vi "Start All Task.vi"(7 "when":timestamp, 8 "error in":errorcluster, 10 "rate":dbl=1000.0 format="%0.2f", 11 "Task in":T1) -> (0 "error out":errorcluster, 3 "Task out":T1)   [LabVIEW 2022 SP3]
uses:
  <vilib>/DAQmx/configure/trigger.llb/DAQmx Start Trigger (Time).vi
  <vilib>/DAQmx/configure/timing.llb/DAQmx Timing (Sample Clock).vi
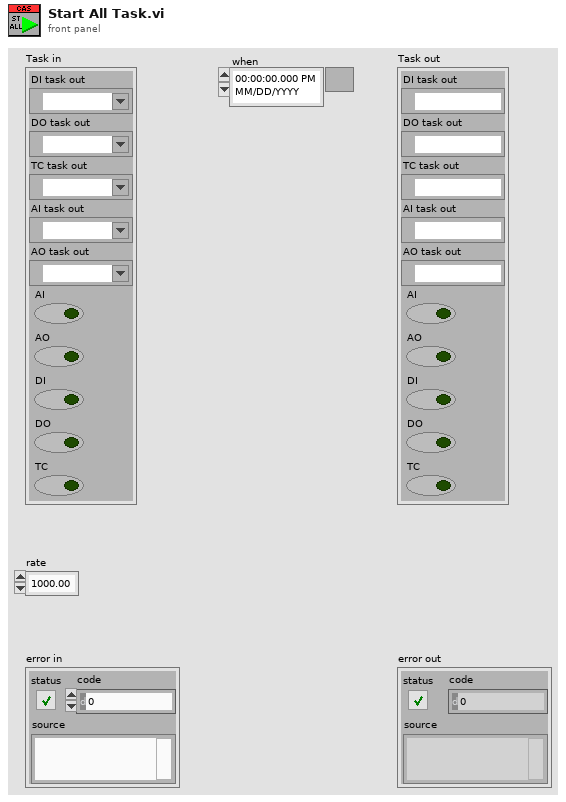
[diagram p1: front panel]
types:
  T1 = cluster{"DI task out":refnum<k21>, "DO task out":refnum<k21>, "TC task out":refnum<k21>, "AI task out":refnum<k21>, "AO task out":refnum<k21>, "AI":bool, "AO":bool, "DI":bool, "DO":bool, "TC":bool}
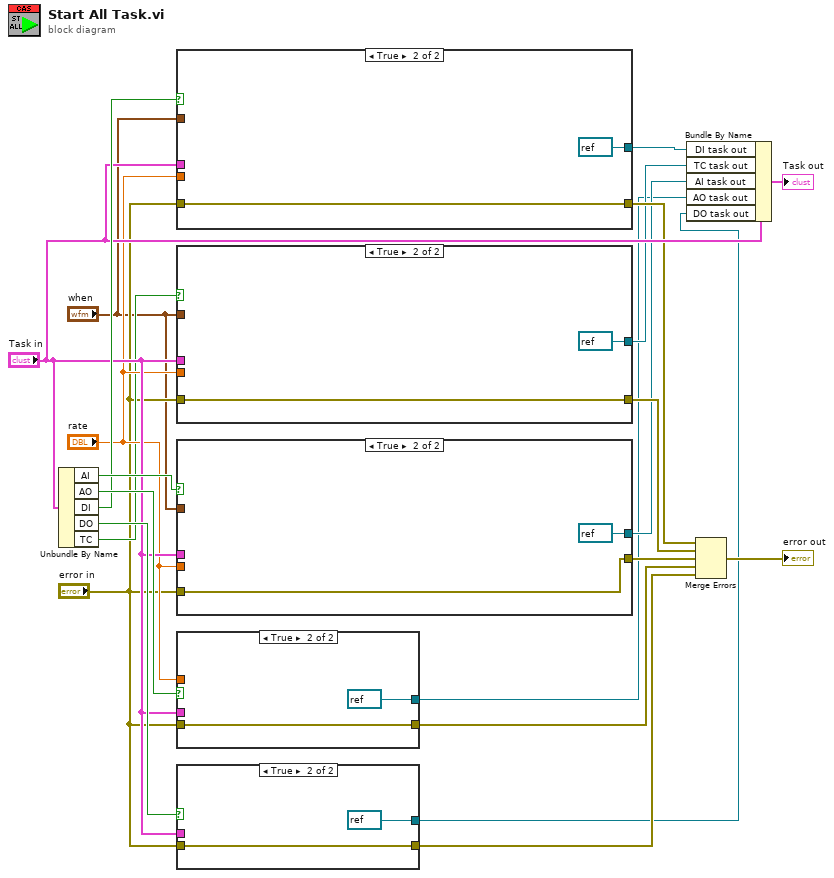
[diagram p0: block diagram]
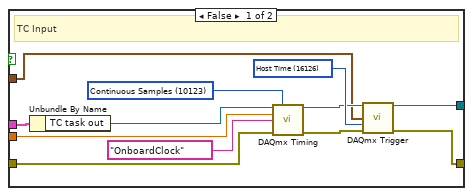
[diagram p2: hidden frame]
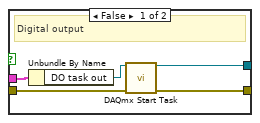
[diagram p3: hidden frame]
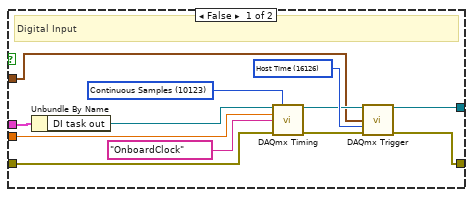
[diagram p4: hidden frame]
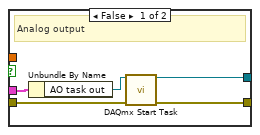
[diagram p5: hidden frame]
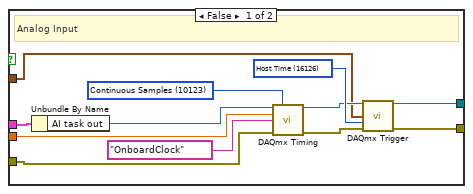
[diagram p6: hidden frame]
diagram:
  n1 = Unbundle By Name("Task in") -> ("AI"=w21:bool, "AO"=w20:bool, "DI"=w19:bool, "DO"=w18:bool, "TC"=w15:bool)
  n2 = case shown="True" w19 {
    tunnel: [w28 w35] -> w13
    tunnel: "rate" -> [w27 _]
    tunnel: "when" -> [w26 _]
    tunnel: "Task in" -> [w23 _]
    tunnel: "error in" -> [w24 w35]
    tunnel: [w22 refnum<k21> refnum ("task out")] -> w7
    frame False {
      w31 = 16126 items=["Host Time"=16126, "I/O Device Time"=16127] ("timescale")
      w32 = 10123 items=["Finite Samples"=10178, "Continuous Samples"=10123, "Hardware Timed Single Point"=12522] ("sample mode")
      # "Digital Input"
      n3 = Unbundle By Name(w23) -> ("DI task out"=w25:refnum<k21>)
      n4 = call-poly <vilib>:"DAQmx Timing.vi"("task/channels in"=w25, "sample mode"=w32, "rate"=w27, "source"=tag "OnboardClock", "error in"=w24) -> ("task out"=w29:refnum<k21>, "error out"=w30:errorcluster)  [unwired: 9 in]
      n5 = call-poly <vilib>:"DAQmx Trigger.vi"("task/channels in"=w29, "when"=w26, "timescale"=w31, "error in"=w30) -> ("task out"=w22:refnum<k21>, "error out"=w28:errorcluster)  [unwired: 10 in]
    }
    frame True {
    }
  }
  n6 = case shown="True" w15 {
    tunnel: "rate" -> [w42 _]
    tunnel: "when" -> [w41 _]
    tunnel: "Task in" -> [w40 _]
    tunnel: "error in" -> [w38 w49]
    tunnel: [w37 w49] -> w12
    tunnel: [w36 refnum<k21> refnum ("task out")] -> w6
    frame False {
      w45 = 16126 items=["Host Time"=16126, "I/O Device Time"=16127] ("timescale")
      w46 = 10123 items=["Finite Samples"=10178, "Continuous Samples"=10123, "Hardware Timed Single Point"=12522] ("sample mode")
      # "TC Input"
      n7 = Unbundle By Name(w40) -> ("TC task out"=w39:refnum<k21>)
      n8 = call-poly <vilib>:"DAQmx Timing.vi"("task/channels in"=w39, "sample mode"=w46, "rate"=w42, "source"=tag "OnboardClock", "error in"=w38) -> ("task out"=w43:refnum<k21>, "error out"=w44:errorcluster)  [unwired: 9 in]
      n9 = call-poly <vilib>:"DAQmx Trigger.vi"("task/channels in"=w43, "when"=w41, "timescale"=w45, "error in"=w44) -> ("task out"=w36:refnum<k21>, "error out"=w37:errorcluster)  [unwired: 10 in]
    }
    frame True {
    }
  }
  n10 = case shown="True" w21 {
    tunnel: [w56 w63] -> w11
    tunnel: "rate" -> [w55 _]
    tunnel: "when" -> [w54 _]
    tunnel: "Task in" -> [w53 _]
    tunnel: "error in" -> [w51 w63]
    tunnel: [w50 refnum<k21> refnum ("task out")] -> w5
    frame False {
      w59 = 16126 items=["Host Time"=16126, "I/O Device Time"=16127] ("timescale")
      w60 = 10123 items=["Finite Samples"=10178, "Continuous Samples"=10123, "Hardware Timed Single Point"=12522] ("sample mode")
      # "Analog Input"
      n11 = Unbundle By Name(w53) -> ("AI task out"=w52:refnum<k21>)
      n12 = call-poly <vilib>:"DAQmx Timing.vi"("task/channels in"=w52, "sample mode"=w60, "rate"=w55, "source"=tag "OnboardClock", "error in"=w51) -> ("task out"=w57:refnum<k21>, "error out"=w58:errorcluster)  [unwired: 9 in]
      n13 = call-poly <vilib>:"DAQmx Trigger.vi"("task/channels in"=w57, "when"=w54, "timescale"=w59, "error in"=w58) -> ("task out"=w50:refnum<k21>, "error out"=w56:errorcluster)  [unwired: 10 in]
    }
    frame True {
    }
  }
  n14 = case shown="True" w20 {
    tunnel: "rate" -> [_ _]
    tunnel: "Task in" -> [w66 _]
    tunnel: "error in" -> [w68 w70]
    tunnel: [w67 w70] -> w10
    tunnel: [w64 refnum<k21> refnum ("task out")] -> w4
    frame False {
      # "Analog output"
      n15 = Unbundle By Name(w66) -> ("AO task out"=w65:refnum<k21>)
      n16 = call <vilib>:"DAQmx Start Task.vi"("task/channels in"=w65, "error in"=w68) -> ("task out"=w64:refnum<k21>, "error out"=w67:errorcluster)  [unwired: 12 in]
    }
    frame True {
    }
  }
  n17 = case shown="True" w18 {
    tunnel: "error in" -> [w75 w77]
    tunnel: [w74 w77] -> w9
    tunnel: "Task in" -> [w72 _]
    tunnel: [w71 refnum<k21> refnum ("task out")] -> w3
    frame False {
      # "Digital output"
      n18 = Unbundle By Name(w72) -> ("DO task out"=w73:refnum<k21>)
      n19 = call <vilib>:"DAQmx Start Task.vi"("task/channels in"=w73, "error in"=w75) -> ("task out"=w71:refnum<k21>, "error out"=w74:errorcluster)  [unwired: 12 in]
    }
    frame True {
    }
  }
  n20 = Bundle By Name(cluster="Task in", "DI task out"=w7, "TC task out"=w6, "AI task out"=w5, "AO task out"=w4, "DO task out"=w3) -> (→"Task out":T1)
  n21 = Merge Errors(w13, w12, w11, w10, w9) -> (→"error out":errorcluster)
